vi "system.lockin_config.vi"(8 "error in (no error)":errorcluster, 10 "runCalculation":T1={"runCalculation"={"adjust gain"=FALSE, "subtract offset"=FALSE, "60 Hz prefilter"=FALSE, "LP prefilter"=FALSE, "lockin"=FALSE, "FFT"=FALSE, "gain"=[], "offset"=[], "LP config"={"high cutoff freq [Hz]"=0.45}, "Lockin config"=[], "FFT config"={"averaging parameters"={"averaging mode"=enum."RMS averaging", "weighting mode"=enum."Exponential", "number of averages"=10}, "window"=1, "export mode"=0, "window parameter"=nan, "restart averaging (F)"=FALSE}}} {"runCalculation"."FFT config"."export mode" items=["Power Spectrum", "Power Spectral Density"]; "runCalculation"."FFT config"."window" items=["Rectangle"=0, "Hanning"=1, "Hamming"=2, "Blackman-Harris"=3, "Exact Blackman"=4, "Blackman"=5, "Flat Top"=6, "4 Term B-Harris "=7, "7 Term B-Harris"=8, "Low Sidelobe"=9, "Blackman Nuttall"=11, "Triangle"=30, "Bartlett-Hanning"=31, "Bohman"=32, "Parzen"=33, "Welch"=34, "Kaiser"=60, "Dolph-Chebyshev"=61, "Gaussian"=62]; "runCalculation"."FFT config"."averaging parameters"."number of averages" min=1; "runCalculation"."Lockin config"."TC (s)" format="%#_13g"}, 11 "lockin":refnum<class "multichannel-lockin.lvclass">) -> (0 "error out":errorcluster, 3 "lockin out":refnum<class "multichannel-lockin.lvclass">)   [LabVIEW 2019, in "multichannel-lockin.lvclass"]
doc: "---------------------------------------------------------------\nJKI State Machine Objects™\nhttp://jki.net/state-machine-objects/\nCopyright (C) 2005-2015, JKI <info@jki.net>\nALL RIGHTS RESERVEDJKI State Machine Objects (SMO) 1.0.0.4\nJKI - JKI\nCopyright (c) 2015, JKI"
uses:
  multichannel-lockin.lvclass
  DSP/Typedefs/LP_Config.ctl
  DSP/DSP.lvclass
  DSP.lockin/Typedefs/Lockin_Config.ctl
  DSP.lockin/DSP_lockin.lvclass
  <vilib>/Analysis/4window.llb/windowTd.ctl
  <vilib>/Analysis/NI_AALPro.lvlib
  <vilib>/measure/maspectr.llb/Power Spectrum and PSD Export Mode.ctl
  <vilib>/measure/NI_MAPro.lvlib
  DSP/Typedefs/FFT_Config.ctl
  DSP/Typedefs/PrivateEvents--DSP.RunCalculation.ctl
panel:
  # "For instructions on how to use the JKI State Machine Objects, examples and video tutorials, visit:\nhttp://jki.net/state-machine-objects/\n\nJKI State Machine Objects™\nhttp://jki.net/state-machine-objects/\nCopyright (C) 2005-2015, JKI <info@jki.net>\nALL RIGHTS RESERVED"
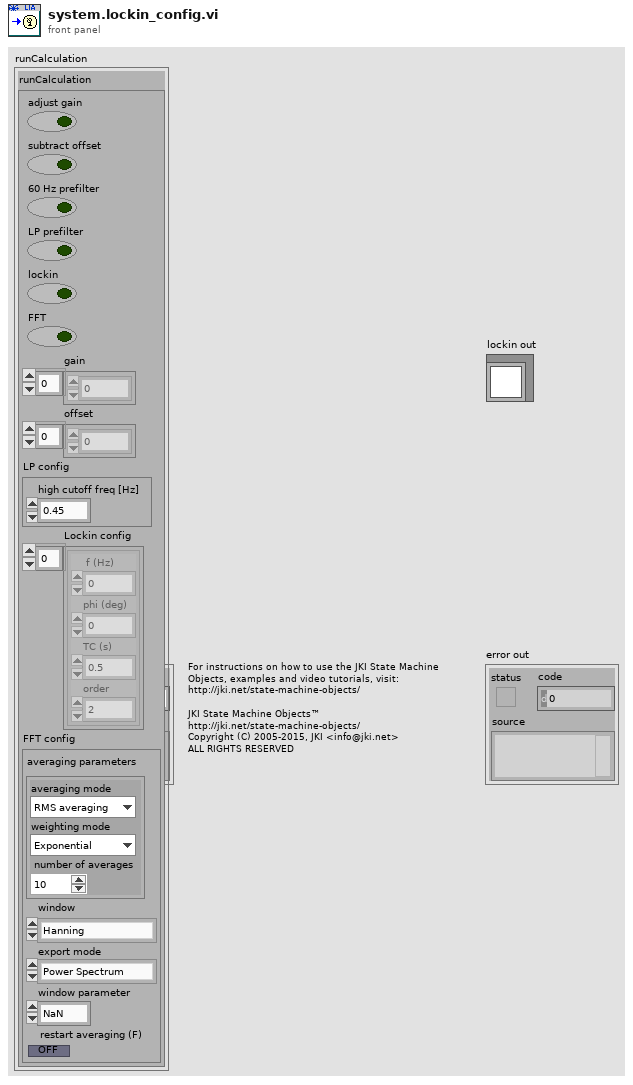
[diagram p1: front panel]
types:
  T1 = typedef "DSP.lvclass/PrivateEvents--DSP.RunCalculation.ctl" = cluster{"runCalculation":cluster{"adjust gain":bool, "subtract offset":bool, "60 Hz prefilter":bool, "LP prefilter":bool, "lockin":bool, "FFT":bool, "gain":dbl[], "offset":dbl[], "LP config":T2, "Lockin config":T3, "FFT config":T4}}
  T2 = typedef "DSP.lvclass/LP_Config.ctl" = cluster{"high cutoff freq [Hz]":dbl}
  T3 = typedef "DSP_lockin.lvclass/Lockin_Config.ctl" = cluster{" f (Hz)":dbl, "phi (deg)":dbl, "TC (s)":dbl, "order":i32}[]
  T4 = typedef "DSP.lvclass/FFT_Config.ctl" = cluster{"averaging parameters":cluster{"averaging mode":enum16{"No averaging", "Vector averaging", "RMS averaging", "Peak hold"}, "weighting mode":enum16{"Linear", "Exponential"}, "number of averages":u32}, "window":T5, "export mode":T6, "window parameter":dbl, "restart averaging (F)":bool}
  T5 = typedef "NI_AALPro.lvlib/windowTd.ctl" = u32
  T6 = typedef "NI_MAPro.lvlib/Power Spectrum and PSD Export Mode.ctl" = u16
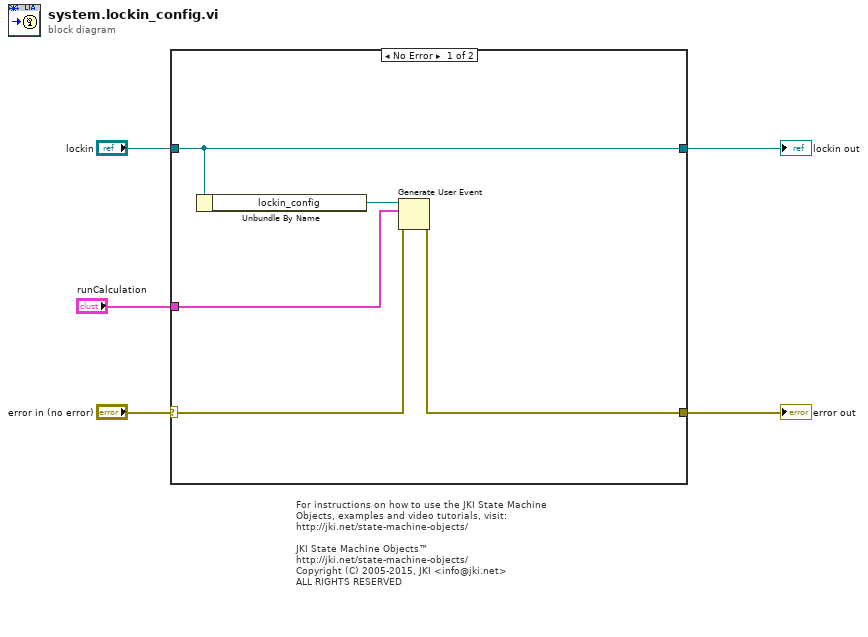
[diagram p0: block diagram]
diagram:
  # "For instructions on how to use the JKI State Machine Objects, examples and video tutorials, visit:\nhttp://jki.net/state-machine-objects/\n\nJKI State Machine Objects™\nhttp://jki.net/state-machine-objects/\nCopyright (C) 2005-2015, JKI <info@jki.net>\nALL RIGHTS RESERVED"
  n1 = case shown="No Error" "error in (no error)" {
    selector: "error in (no error)" -> [w10 w12]
    tunnel: [w8 w12] -> w4
    tunnel: [w7 w11] -> w5
    tunnel: "lockin" -> [w7 w11]
    tunnel: "runCalculation" -> [w6 _]
    frame No Error {
      n2 = Unbundle By Name(w7) -> ("lockin_config"=w9:refnum<user-event>)
      n3 = Generate User Event(user event=w9, event data cluster=w6, error in=w10) -> (error out=w8:errorcluster)  [unwired: 1 in, 1 out]
    }
    frame Error {
    }
  }
  "error out" <- w4
  "lockin out" <- w5
